vi "H036 Harsh Pandit SCADA Lab 3a Sem 6.vi"() -> ()   [LabVIEW 2018]
panel:
  in  "Input 2":bool
  in  "Input 1":bool
  out "Carry":bool
  out "Sum":bool
  # "Experiment 3a: Develop half adder as a sub VI"
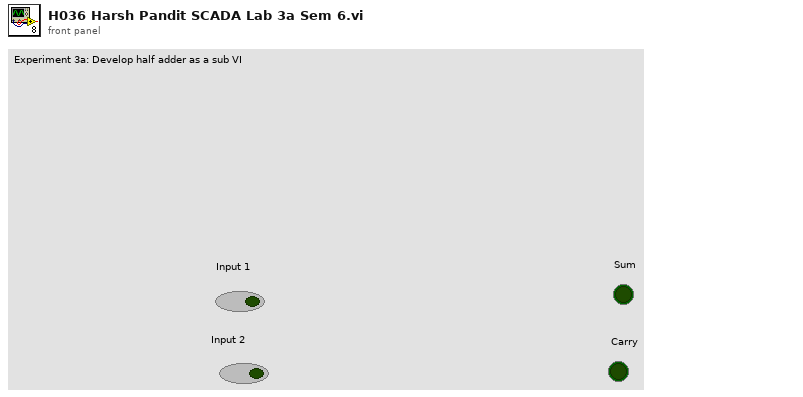
[diagram p1: front panel]
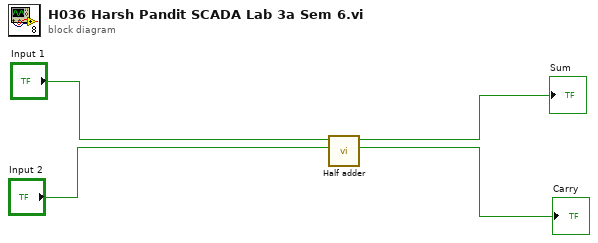
[diagram p0: block diagram]
diagram:
  n1 = call "Half adder.vi"("Input in"="Input 2", "Input 1"="Input 1") -> ("Boolean"=→"Carry":bool, "Boolean 2"=→"Sum":bool)  [unwired: 8 in]
